vi "Close.vi"(8 "error in":errorcluster, 11 "Cycler Cluster - 24 Channel.lvclass":refnum<class "Cycler Cluster - 24 Channel.lvclass">) -> (0 "error out":errorcluster)   [LabVIEW 2023, in "Cycler Cluster - 24 Channel.lvclass"]
uses:
  Cycler Cluster - 24 Channel.lvclass
  Cycler Cluster - 24 Channel.lvclass/Cycler Cluster - 24 Channel.ctl
  <vilib>/ADAS Replay HIL/AdasHilServices/AdasHilServices Fill In Error Info Ex.vi
  <vilib>/ADAS Replay HIL/AdasHilServices/AdasHilChannelServices.lvlib
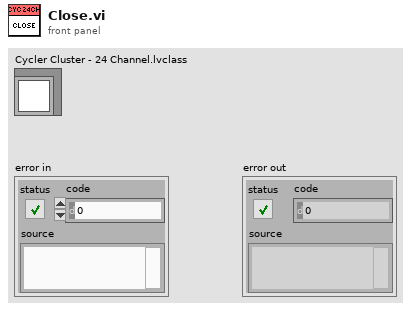
[diagram p1: front panel]
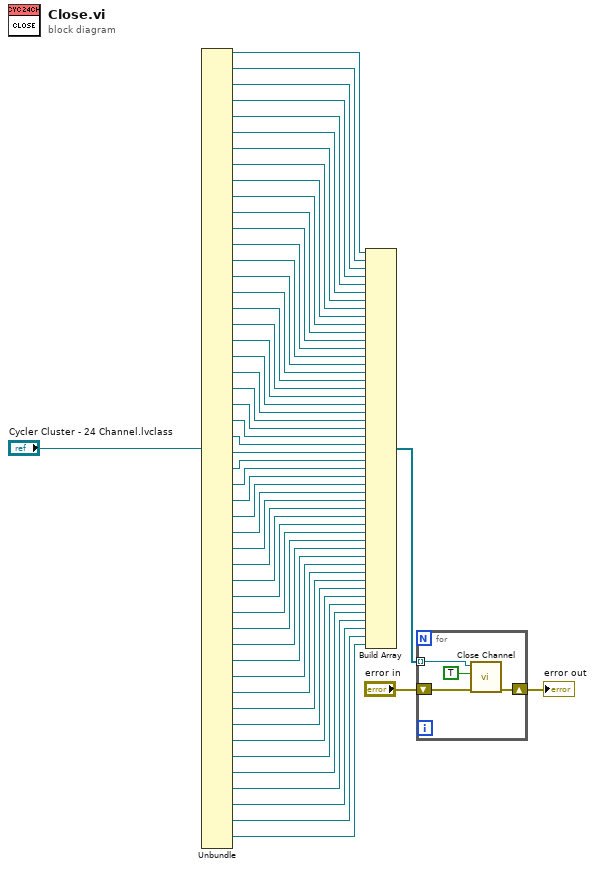
[diagram p0: block diagram]
diagram:
  n1 = Unbundle("Cycler Cluster - 24 Channel.lvclass") -> (w53:refnum<k21>, w52:refnum<k21>, w48:refnum<k21>, w47:refnum<k21>, w46:refnum<k21>, w45:refnum<k21>, w44:refnum<k21>, w43:refnum<k21>, w42:refnum<k21>, w41:refnum<k21>, w40:refnum<k21>, w39:refnum<k21>, w38:refnum<k21>, w37:refnum<k21>, w36:refnum<k21>, w35:refnum<k21>, w34:refnum<k21>, w33:refnum<k21>, w32:refnum<k21>, w31:refnum<k21>, w30:refnum<k21>, w29:refnum<k21>, w28:refnum<k21>, w27:refnum<k21>, w26:refnum<k21>, w25:refnum<k21>, w24:refnum<k21>, w23:refnum<k21>, w22:refnum<k21>, w21:refnum<k21>, w20:refnum<k21>, w19:refnum<k21>, w18:refnum<k21>, w17:refnum<k21>, w16:refnum<k21>, w15:refnum<k21>, w14:refnum<k21>, w13:refnum<k21>, w12:refnum<k21>, w11:refnum<k21>, w10:refnum<k21>, w9:refnum<k21>, w8:refnum<k21>, w7:refnum<k21>, w6:refnum<k21>, w5:refnum<k21>, w4:refnum<k21>, w3:refnum<k21>, w2:refnum<k21>, w1:refnum<k21>)  [unwired: 50 out]
  n2 = Build Array(w53, w52, w48, w47, w46, w45, w44, w43, w42, w41, w40, w39, w38, w37, w36, w35, w34, w33, w32, w31, w30, w29, w28, w27, w26, w25, w24, w23, w22, w21, w20, w19, w18, w17, w16, w15, w14, w13, w12, w11, w10, w9, w8, w7, w6, w5, w4, w3, w2, w1) -> (w51:refnum<k21>[])
  n3 = for {
    tunnel: w51 -> [w58] mode=indexing
    shift-right: [w55] -> w49
    shift-left: "error in" -> [w56]
    n4 = call <vilib>:"Close Channel.vi"("error in"=w56, "Force Destroy? (F)"=TRUE, "ADAS HIL Channel"=w58) -> ("error out"=w55:errorcluster)  [unwired: 8 in]
  }
  "error out" <- w49
